vi "TCPopenConnection.vi"(0 "DashboardServer in":refnum<class "Dashboard Server.lvclass">, 5 "error in (no error)":errorcluster) -> (14 "DashboardServer out":refnum<class "Dashboard Server.lvclass">, 15 "connectionStatus":string, 16 "connected":bool, 19 "error out":errorcluster)   [LabVIEW 2016, in "Dashboard Server.lvclass"]
uses:
  Dashboard Server.lvclass
  Dashboard Server.lvclass/Dashboard Server.ctl
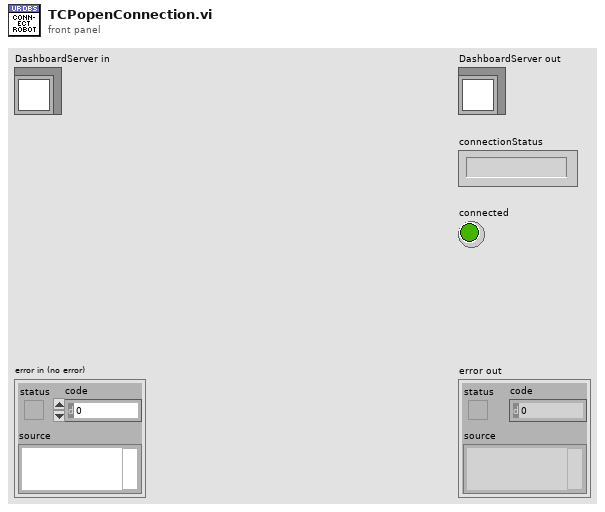
[diagram p1: front panel]
types:
  T1 = enum16{"Standard", "Buffered", "CRLF", "Immediate"}
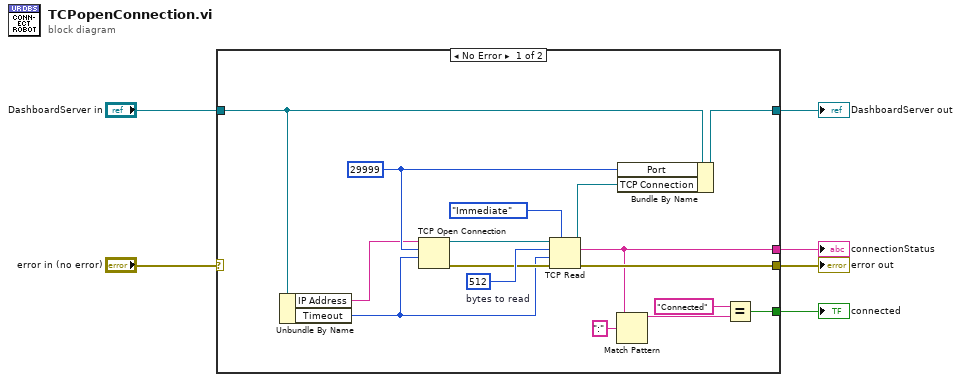
[diagram p0: block diagram]
diagram:
  n1 = case shown="No Error" "error in (no error)" {
    selector: "error in (no error)" -> [_ w24]
    tunnel: [w15 w24] -> w5
    tunnel: [w16 w23] -> w3
    tunnel: "DashboardServer in" -> [w14 w23]
    tunnel: [w12 _] -> w2
    tunnel: [w8 _] -> w1
    frame No Error {
      w20 = u16 29999 ("remote port or service name")
      w21 = 512  # bytes to read
      n2 = Unbundle By Name(w14) -> ("IP Address"=w7:string, "Timeout"=w13:i32)
      n3 = TCP Open Connection(address=w7, remote port or service name=w20, timeout ms (60000)=w13) -> (connection ID=w18:refnum<k5>, error out=w19:errorcluster)  [unwired: 2 in]
      n4 = TCP Read(connection ID=w18, bytes to read=w21, error in (no error)=w19, 7:T1."Immediate" ("mode (standard)"), 9:w13) -> (connection ID out=w17:refnum<k5>, data out=w12:string, error out=w15:errorcluster)
      n5 = Match Pattern(string=w12, regular expression=":") -> (before substring=w10:string)  [unwired: 1 in, 3 out]
      n6 = Bundle By Name(cluster=w14, "Port"=w20, "TCP Connection"=w17) -> (w16:refnum<class "Dashboard Server.lvclass">)
      n7 = Equal?(x="Connected", y=w10) -> (x = y?=w8:bool)
    }
    frame Error {
    }
  }
  "error out" <- w5
  "DashboardServer out" <- w3
  "connectionStatus" <- w2
  "connected" <- w1
